vi "Actor Core.vi"(8 "error in":errorcluster, 11 "State in":refnum<class "Command.lvclass">) -> (0 "error out":errorcluster, 3 "Actor out":refnum<class "Actor.lvclass">)   [LabVIEW 2013, in "Command Processor.lvlib" / "Command.lvlib" / "Command.lvclass"]
doc: "(<B>Filename</B>: Actor Framework.lvlib:Actor.lvclass:Actor Core.vi)\n\nThis override invokes Entry.vi on the initial state, prior to calling the parent Actor Core. Adding this behavior to Actor Core (instead of an override of Pre Launch Init.vi) allows the initial state to launch a nested actor as part of its entry behavior.\n\nReceives messages to the actor, reacts to them, and initiates any error handling that may shut the actor down.\n\nDescendant classes may override this VI to append parallel tasks for the actor to complete while it handles messages. Overrides use the Call Parent Method node."
uses:
  Command.lvclass
  <vilib>/ni/Actors/State Actor/State Actor/State Actor.lvclass
  <vilib>/ActorFramework/Actor/Actor.lvclass
  State Status.ctl
  Command Status.ctl
panel:
  in  "Command Status":T1
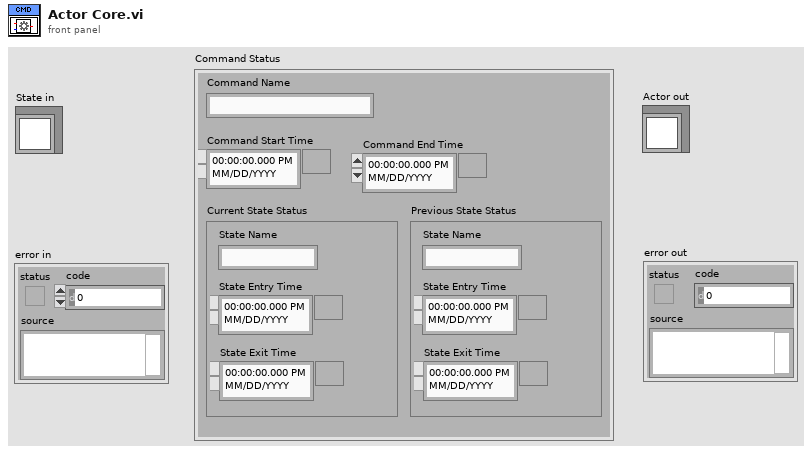
[diagram p1: front panel]
types:
  T1 = typedef "Command Processor.lvlib/Command.lvlib/Command.lvclass/Command Status.ctl" = cluster{"Command Name":string, "Current State Status":T2, "Command Start Time":timestamp, "Command End Time":timestamp, "Previous State Status":T2}
  T2 = typedef "Command Processor.lvlib/Command.lvlib/Command.lvclass/State Status.ctl" = cluster{"State Name":string, "State Entry Time":timestamp, "State Exit Time":timestamp}
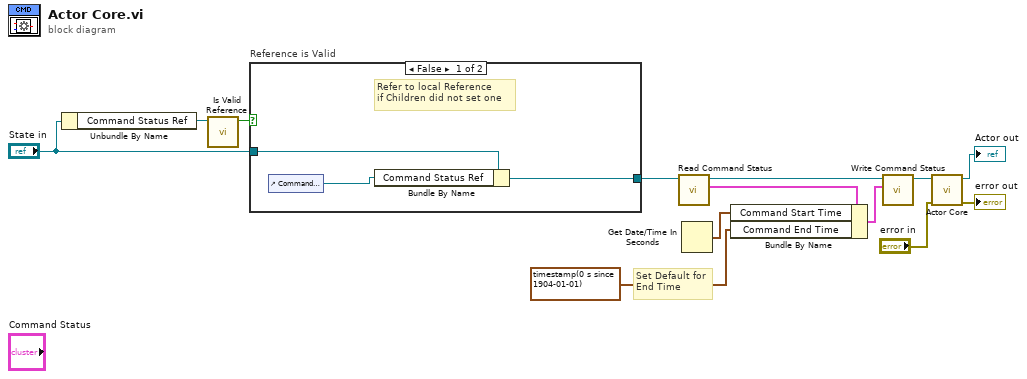
[diagram p0: block diagram]
diagram:
  # "Set Default for\nEnd Time"
  n1 = Unbundle By Name("State in") -> ("Command Status Ref"=w10:refnum<vi>)
  n2 = call "Is Valid Reference.vi"("Reference"=w10) -> ("Reference Is Valid"=w9:bool)  [unwired: 10 in]
  n3 = case "Reference is Valid" shown="False" w9 {
    tunnel: "State in" -> [w16 w17]
    tunnel: [w14 w17] -> w2
    frame False {
      # "Refer to local Reference\nif Children did not set one"
      n4 = control-ref of="Command Status"() -> (w15:refnum<vi>)
      n5 = Bundle By Name(cluster=w16, "Command Status Ref"=w15) -> (w14:refnum<class "Command.lvclass">)
    }
    frame True {
    }
  }
  n6 = call-dynamic "Read Command Status.vi"("Command in"=w2) -> ("Command Status"=w4:T1, "Command out"=w3:refnum<class "Command.lvclass">)  [unwired: 8 in, 1 out]
  n7 = Get Date/Time In Seconds() -> (seconds since 1Jan1904=w6:timestamp)
  n8 = Bundle By Name(cluster=w4, "Command Start Time"=w6, "Command End Time"=timestamp(0 s since 1904-01-01)) -> (w5:T1)
  n9 = call-dynamic "Write Command Status.vi"("Command Status"=w5, "Command in"=w3) -> ("Command out"=w1:refnum<class "Command.lvclass">)  [unwired: 8 in, 1 out]
  n10 = call-parent "Actor Core.vi"("error in"="error in", "State in"=w1) -> ("error out"=→"error out":errorcluster, "Actor out"=→"Actor out":refnum<class "Actor.lvclass">)  [unwired: 8 in]
